vi "Initialize NI-SWITCH Custom Device.vi"(8 "error in":errorcluster, 11 "ni-switch custom device in":T1 format="%.0x") -> (0 "error out":errorcluster, 2 "endpoint configuration section":T1 format="%.0x", 3 "ni-switch custom device out":T1 format="%.0x")   [LabVIEW 2019, in "NI-SWITCH Scripting.lvlib"]
uses:
  NI-SWITCH Scripting.lvlib
  <vilib>/NI VeriStand/Custom Device API/Custom Device Item Ref.ctl
  Properties/NI-SWITCH All Properties.ctl
  NI-SWITCH Constants.vi
  Shared/Constants.vi
  <vilib>/NI VeriStand/Custom Device API/Custom Device API.lvlib
  Shared/NI-SWITCH Shared.lvlib
  Shared/Routing and Faulting Hardware API/Routing and Faulting Hardware API.lvlib
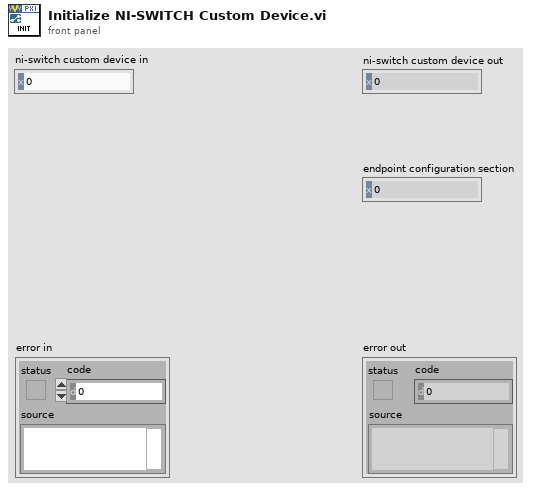
[diagram p1: front panel]
types:
  T1 = typedef "Custom Device API.lvlib/Custom Device Item Ref.ctl" = u64
  T2 = typedef "NI-SWITCH Scripting.lvlib/NI-SWITCH All Properties.ctl" = cluster{"Resource":string, "Topology":string, "Description":string}
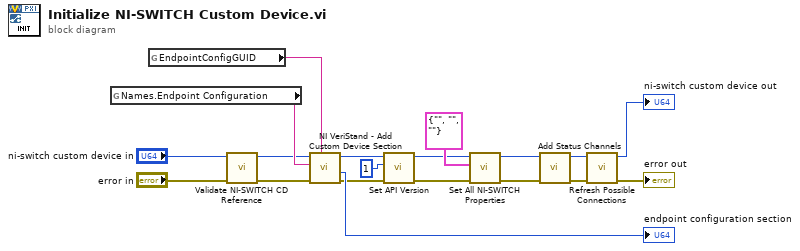
[diagram p0: block diagram]
diagram:
  n1 = global read "NI-SWITCH Constants.vi" "Names.Endpoint Configuration"() -> (w18:string)
  n2 = global read "Constants.vi" "EndpointConfigGUID"() -> (w15:string)
  n3 = call "Validate NI-SWITCH CD Reference.vi"("error in"="error in", "ni-switch custom device in"="ni-switch custom device in") -> ("error out"=w7:errorcluster, "ni-switch custom device out"=w5:T1)  [unwired: 8 in]
  n4 = call <vilib>:"NI VeriStand - Add Custom Device Section.vi"("GUID (Default Section)"=w15, "error in (no error)"=w7, "Section Name"=w18, "Parent Ref in"=w5) -> ("error out"=w11:errorcluster, "Section Ptr"=→"endpoint configuration section":T1, "Parent Ref out"=w12:T1)  [unwired: 4 in, 1 out]
  n5 = call "Set API Version.vi"("error in (no error)"=w11, "API version"=u32 1, "Hardware Ref in"=w12) -> ("error out"=w10:errorcluster, "Hardware Ref out"=w9:T1)  [unwired: 7 in]
  n6 = call "Set All NI-SWITCH Properties.vi"("error in"=w10, "properties"=T2 {"Resource"="", "Topology"="", "Description"=""} ("SLSC Switch All Properties"), "ni-switch custom device in"=w9) -> ("error out"=w14:errorcluster, "ni-switch custom device out"=w13:T1)  [unwired: 7 in]
  n7 = call "Add Status Channels.vi"("error in"=w14, "ni-switch custom device in"=w13) -> ("error out"=w4:errorcluster, "ni-switch custom device out"=w3:T1)  [unwired: 8 in]
  n8 = call "Refresh Possible Connections.vi"("error in"=w4, "ni-switch custom device in"=w3) -> ("error out"=→"error out":errorcluster, "ni-switch custom device out"=→"ni-switch custom device out":T1)  [unwired: 8 in]
